vi "Write Tag.vi"(8 "error in (no error)":errorcluster, 10 "Tag":string, 11 "bt_Blackboard_Leaf Type in":refnum<class "bt_Blackboard_Leaf Type.lvclass">) -> (0 "error out":errorcluster, 3 "bt_Blackboard_Leaf Type out":refnum<class "bt_Blackboard_Leaf Type.lvclass">)   [LabVIEW 2021, in "BT.lvlib" / "bt_Blackboard_Leaf Type.lvclass"]
uses:
  bt_Blackboard_Leaf Type.lvclass
  bt_Blackboard_Leaf Type.lvclass/bt_Blackboard_Leaf Type.ctl
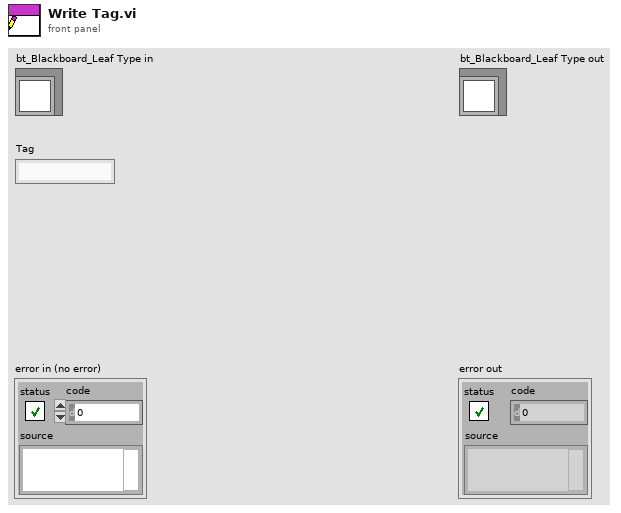
[diagram p1: front panel]
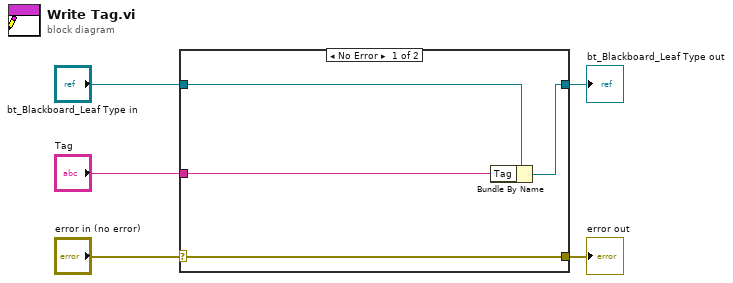
[diagram p0: block diagram]
diagram:
  n1 = case shown="No Error" "error in (no error)" {
    selector: "error in (no error)" -> [w9 w10]
    tunnel: [w9 w10] -> w4
    tunnel: [w7 w11] -> w2
    tunnel: "bt_Blackboard_Leaf Type in" -> [w8 w11]
    tunnel: "Tag" -> [w6 _]
    frame No Error {
      n2 = Bundle By Name(cluster=w8, "Tag"=w6) -> (w7:refnum<class "bt_Blackboard_Leaf Type.lvclass">)
    }
    frame Error {
    }
  }
  "error out" <- w4
  "bt_Blackboard_Leaf Type out" <- w2
